vi "DAQ_Static Dig Meas Initialize.vi"(0 "Physical Channels":tag, 7 "Global Channels":refnum<k21>, 11 "error in":errorcluster) -> (4 "DAQmx Task Out":refnum<k21>, 15 "error out":errorcluster)   [LabVIEW 2021, in "DAQ_Static Digital State Measurement.lvlib"]
doc: "Initialize Digital Input channels and obtains a DAQmx task\n\nProvide either Physical channel or Global Channel. If both physical and Global channels are provided, Global Channels will take precedence.\n\n<B>Note:</B> This Library supports only digital line in the physical/global channel. <B>Port</B> is <B>not supported</B> in this library and returns an error. User can either use <B>Dynamic Digital Pattern Measurement Library</B> to support port based inputs or specify the ports in line based format (Ex: <B>DIO/port0/line0:31</B>) with the current library."
uses:
  DAQ_Static Digital State Measurement.lvlib
  <vilib>/DAQmx/create/channels.llb/DAQmx Create Channel (DI-Digital Input).vi
panel:
  # "Inputs"
  # "Outputs"
  # "Overview:\nThis VI initializes Digital input channels for static digital measurements and provides the DAQmx Task Out\n\nHardware Requirement: A compatible PXI, PCIe, USB, cDAQ or Testscale device\n\nSoftware Requirement: NI DAQmx 2022Q4 or later\n\nInstructions:\n1. Enter physical channel in which Static Digital State Measurement has to be done in Physical Channels control. (Or) Enter Global channels to use it instead of initiating a new task. User must configure only one input. If both are provided, Global Channels will take precedence.\n2. Get the Digital Measurement task from DAQmx Task Out which stores the reference to the virtual digital input channels.\n\nNotes: \n1. User can use the DAQmx Task on other VI in this library to configure and initiate Static Digital State Measurement task. \n2. This Library supports only digital line in the physical/global channel. Port is not supported in this library and returns an error. User can either use Dynamic Digital Pattern Measurement Library to support port based inputs or specify the ports in line based format (Ex: DIO/port0/line0:31) with the current library."
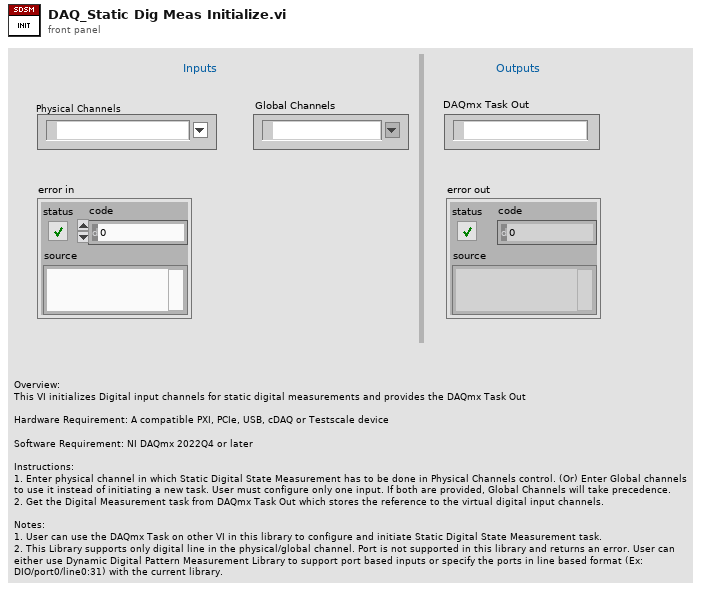
[diagram p1: front panel]
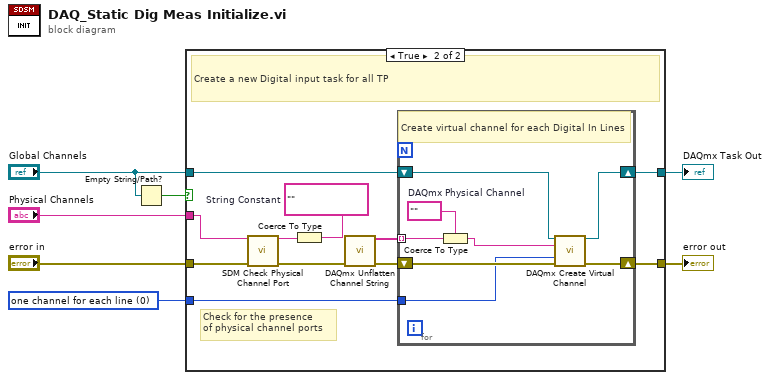
[diagram p0: block diagram]
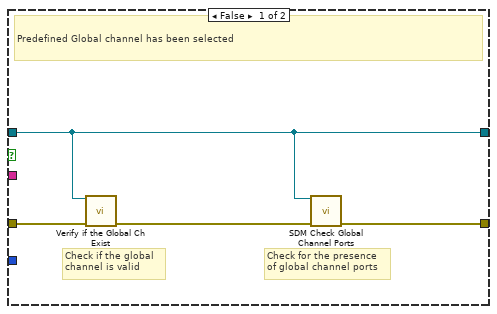
[diagram p2: hidden frame]
diagram:
  w1 = 0 items=["one channel for each line", "one channel for all lines"] ("line grouping")
  n1 = Empty String/Path?(string/path="Global Channels") -> (empty?=w2:bool)
  n2 = case shown="True" w2 {
    tunnel: "Physical Channels" -> [_ w16]
    tunnel: "Global Channels" -> [w11 w18]
    tunnel: [w11 w22] -> w4
    tunnel: "error in" -> [w10 w17]
    tunnel: [w8 w21] -> w7
    tunnel: w1 -> [_ w23]
    frame False {
      # "Check for the presence\nof global channel ports"
      # "Check if the global\nchannel is valid"
      # "Predefined Global channel has been selected"
      n3 = call "Verify if the Global Ch Exist.vi"("Global Channels"=w11, "error in (no error)"=w10) -> ("error out"=w9:errorcluster)  [unwired: 13 in]
      n4 = call "SDM Check Global Channel Ports.vi"("Global Channel In"=w11, "error in (no error)"=w9) -> ("error out"=w8:errorcluster)  [unwired: 12 in, 1 out]
    }
    frame True {
      w13 = ""  # String Constant
      # "Check for the presence \nof physical channel ports"
      # "Create a new Digital input task for all TP"
      n5 = call "SDM Check Physical Channel Port.vi"("Physical Channel In"=w16, "error in (no error)"=w17) -> ("Physical Channel Out"=w14:tag, "error out"=w15:errorcluster)  [unwired: 12 in]
      n6 = Coerce To Type(0:w14, 1:w13) -> (2:w12:string)
      n7 = call <vilib>:"DAQmx Unflatten Channel String.vi"("names in"=w12, "error in"=w15) -> ("names out"=w19:string[], "error out"=w20:errorcluster)  [unwired: 12 in]
      n8 = for {
        shift-right: [w30] -> w22
        shift-left: w18 -> [w31]
        shift-right: [w28] -> w21
        shift-left: w20 -> [w29]
        tunnel: w19 -> [w25] mode=indexing
        tunnel: w23 -> [w27]
        w26 = tag ""  # DAQmx Physical Channel
        # "Create virtual channel for each Digital In Lines"
        n9 = Coerce To Type(0:w25, 1:w26) -> (2:w24:tag)
        n10 = call-poly <vilib>:"DAQmx Create Virtual Channel.vi"("task in"=w31, "lines"=w24, "line grouping"=w27, "error in"=w29) -> ("task out"=w30:refnum<k21>, "error out"=w28:errorcluster)  [unwired: 10 in]
      }
    }
  }
  "DAQmx Task Out" <- w4
  "error out" <- w7
